vi "Data Recorder.vi"() -> ()   [LabVIEW 2021]
uses:
  Type Definitions/Data Frame.ctl
  Type Definitions/Data Frame Header.ctl
  Type Definitions/Payload Class.ctl
  Type Definitions/Device.ctl
  Type Definitions/Real Time Task Status.ctl
  Type Definitions/Enum - Data.ctl
  <vilib>/Platform/TimedLoop/XDataNode/timing_clust.ctl
  <vilib>/Platform/TimedLoop/XDataNode/nitl_modes.ctl
  <vilib>/Platform/TimedLoop/XDataNode/wakeup.ctl
  Type Definitions/Analog Data.ctl
  Type Definitions/Digital Input Data.ctl
  Type Definitions/Internet Connection Monitor.ctl
  Type Definitions/CPU Usage.ctl
  Type Definitions/Telemetry Recorder Status.ctl
  Type Definitions/Memory Monitor.ctl
  Type Definitions/Queue Monitor.ctl
  Type Definitions/RTOSMonitor.ctl
  Type Definitions/System Time.ctl
  <vilib>/platform/TimedLoop/XDataNode/XDataNode.xnode
  <vilib>/Platform/TimedLoop/XDataNode/XDNodeRunTimeDep.lvlib
panel:
  out "Frame":T1 {"CRC" format="%08x"; "Frame Header"."Options" format="%016b"; "Frame Header"."Time" format="%^<%I:%M:%S%3u %p\n%m/%d/%Y %Z>T"; "Frame Header"."Sync" format="%08x"}
  out "Payload ID":u16
  out "Numeric 2":i32
  out "error out 6":errorcluster
  out "Unhandled Data":T1 {"CRC" format="%08x"; "Frame Header"."Options" format="%016b"; "Frame Header"."Time" format="%^<%I:%M:%S%3u %p\n%m/%d/%Y %Z>T"; "Frame Header"."Sync" format="%08x"}
  out "error out 5":errorcluster
  out "error out 4":errorcluster
  out "error out 3":errorcluster
  out "error out 2":errorcluster
  out "output cluster":T5={"Task Name"="", "Priority"=100, "Processor"=-2, "Offset"=0, "Iteration Duration"=0, "Period"=0, "Finished Late"=FALSE}
  out "Numeric":i32
  out "error out":errorcluster
  out "data":T1 {"CRC" format="%08x"; "Frame Header"."Options" format="%016b"; "Frame Header"."Time" format="%^<%I:%M:%S%3u %p\n%m/%d/%Y %Z>T"; "Frame Header"."Sync" format="%08x"}
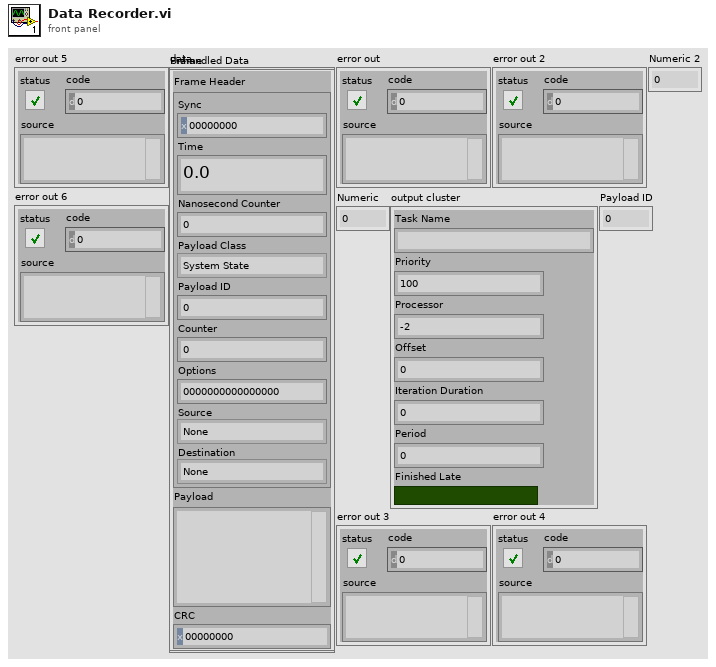
[diagram p1: front panel]
types:
  T1 = typedef "Data Frame.ctl" = cluster{"Frame Header":T2, "Payload":string, "CRC":u32}
  T2 = typedef "Data Frame Header.ctl" = cluster{"Sync":u32, "Time":dbl, "Nanosecond Counter":i64, "Payload Class":T3, "Payload ID":u16, "Counter":i32, "Options":u32, "Source":T4, "Destination":T4}
  T3 = typedef "Payload Class.ctl" = enum16{"System State", "Parameters", "Metadata", "Software Monitor", "Data", "Commands"}
  T4 = typedef "Device.ctl" = enum32{"None", "Exec", "Aux1", "Aux2", "Aux3"}
  T5 = typedef "Real Time Task Status.ctl" = cluster{"Task Name":string, "Priority":i32, "Processor":i32, "Offset":i64, "Iteration Duration":i64, "Period":i64, "Finished Late":bool}
  T6 = typedef "Enum - Data.ctl" = enum16{"Analog Input Data", "Notification Data", "Analog Output Data", "Digital Output Data", "Command Ack", "Digital Input Data", "GPS Solution Data"}
  T7 = enum16{"open", "replace", "create", "open or create", "replace or create", "replace or create with confirmation"}
  T8 = typedef "XDNodeRunTimeDep.lvlib/timing_clust.ctl" = cluster{"Expected End [f-1]":u64, "Actual End [f-1]":u64, "Finished Late? [f-1]":bool, "Expected End [i-1]":u64, "Actual End [i-1]":u64, "Finished Late? [i-1]":bool, "Expected Start [i]":u64, "Actual Start [i]":u64, "Expected Start [f]":u64, "Actual Start [f]":u64, "Source Name":string, "Structure Name":string, "Period":i64, "Deadline":i64, "Offset":i64, "Start":i64, "Priority":i32, "Timeout":i32, "Mode":T9, "Wakeup Reason":T10, "Error":errorcluster, "Source Type":string, "Secondary Source Type":string, "Global End Time":u64, "Global Start Time":u64, "Frame Duration":u64, "Iteration Duration":u64, "Assigned CPU":i32, "I/O Scan Engine Mode":u32}
  T9 = typedef "XDNodeRunTimeDep.lvlib/nitl_modes.ctl" = enum32{"No Change", "Process missed periods, maintain original phase", "Discard missed periods, maintain original phase", "Process missed periods, ignore original phase", "Discard missed periods, ignore original phase"}
  T10 = typedef "XDNodeRunTimeDep.lvlib/wakeup.ctl" = enum32{"Normal", "Aborted", "Asynchronous wakeup", "Timing source error", "Timed loop error", "Timeout"}
  T11 = typedef "Analog Data.ctl" = cluster{"Analog Data":sgl[][]}
  T12 = typedef "Digital Input Data.ctl" = cluster{"Digital Data":u64[][]}
  T13 = typedef "Internet Connection Monitor.ctl" = cluster{"Connected?":bool, "Ping Latency (uS)":i32, "Ping Address":string}
  T14 = typedef "CPU Usage.ctl" = cluster{"User CPU Usage":sgl, "System CPU Usage":sgl, "NIC CPU ":sgl, "IO CPU Usage":sgl, "IRQ CPU Usage":sgl, "SIRQ CPU Usage":sgl, "Idle CPU Time":sgl}
  T15 = typedef "Telemetry Recorder Status.ctl" = cluster{"Filepath":string, "File Size":i64, "Frame Count":i32, "Mean MB/hour":sgl}
  T16 = typedef "Memory Monitor.ctl" = cluster{"Total Memory":sgl, "Available Memory":sgl}
  T17 = typedef "Queue Monitor.ctl" = cluster{"Queue Name":string, "Max Queue Size":i32, "Pending Remove":i32, "Pending Insert":i32, "Elements in Queue":i32}
  T18 = typedef "RTOSMonitor.ctl" = cluster{"Task Name":string, "Priority":i32, "Processor":i32, "Offset":i64, "Min Duration":i64, "Mean Duration":i64, "Max Duration":i64, "Period":i64, "Late Iterations":i16, "Iteration Count":i32}
  T19 = typedef "System Time.ctl" = cluster{"System Clock":timestamp, "GPS Clock":timestamp, "Nanosecond Counter":i64, "GPS Status":enum8{"Initializing", "Normal", "Unable to get fix"}, "GPS Antenna Status":enum8{"Unknown", "Normal", "Absent", "Overcurrent"}, "GPS Satelites Available":u8, "GPS Time (ns)":u64, "GPS UTC Offset":i8, "GPS Time Offset":i32, "UTC Offset Valid":bool, "GPS Time Lock":bool}
  T20 = typedef "LVDateTimeRec.ctl" = cluster{"fractional second":dbl, "second":i32, "minute":i32, "hour":i32, "day of month":i32, "month":i32, "year":i32, "day of week":i32, "day of year":i32, "DST":i32}
  T21 = enum8{"Initializing", "Normal", "Unable to get fix"}
  T22 = enum8{"Unknown", "Normal", "Absent", "Overcurrent"}
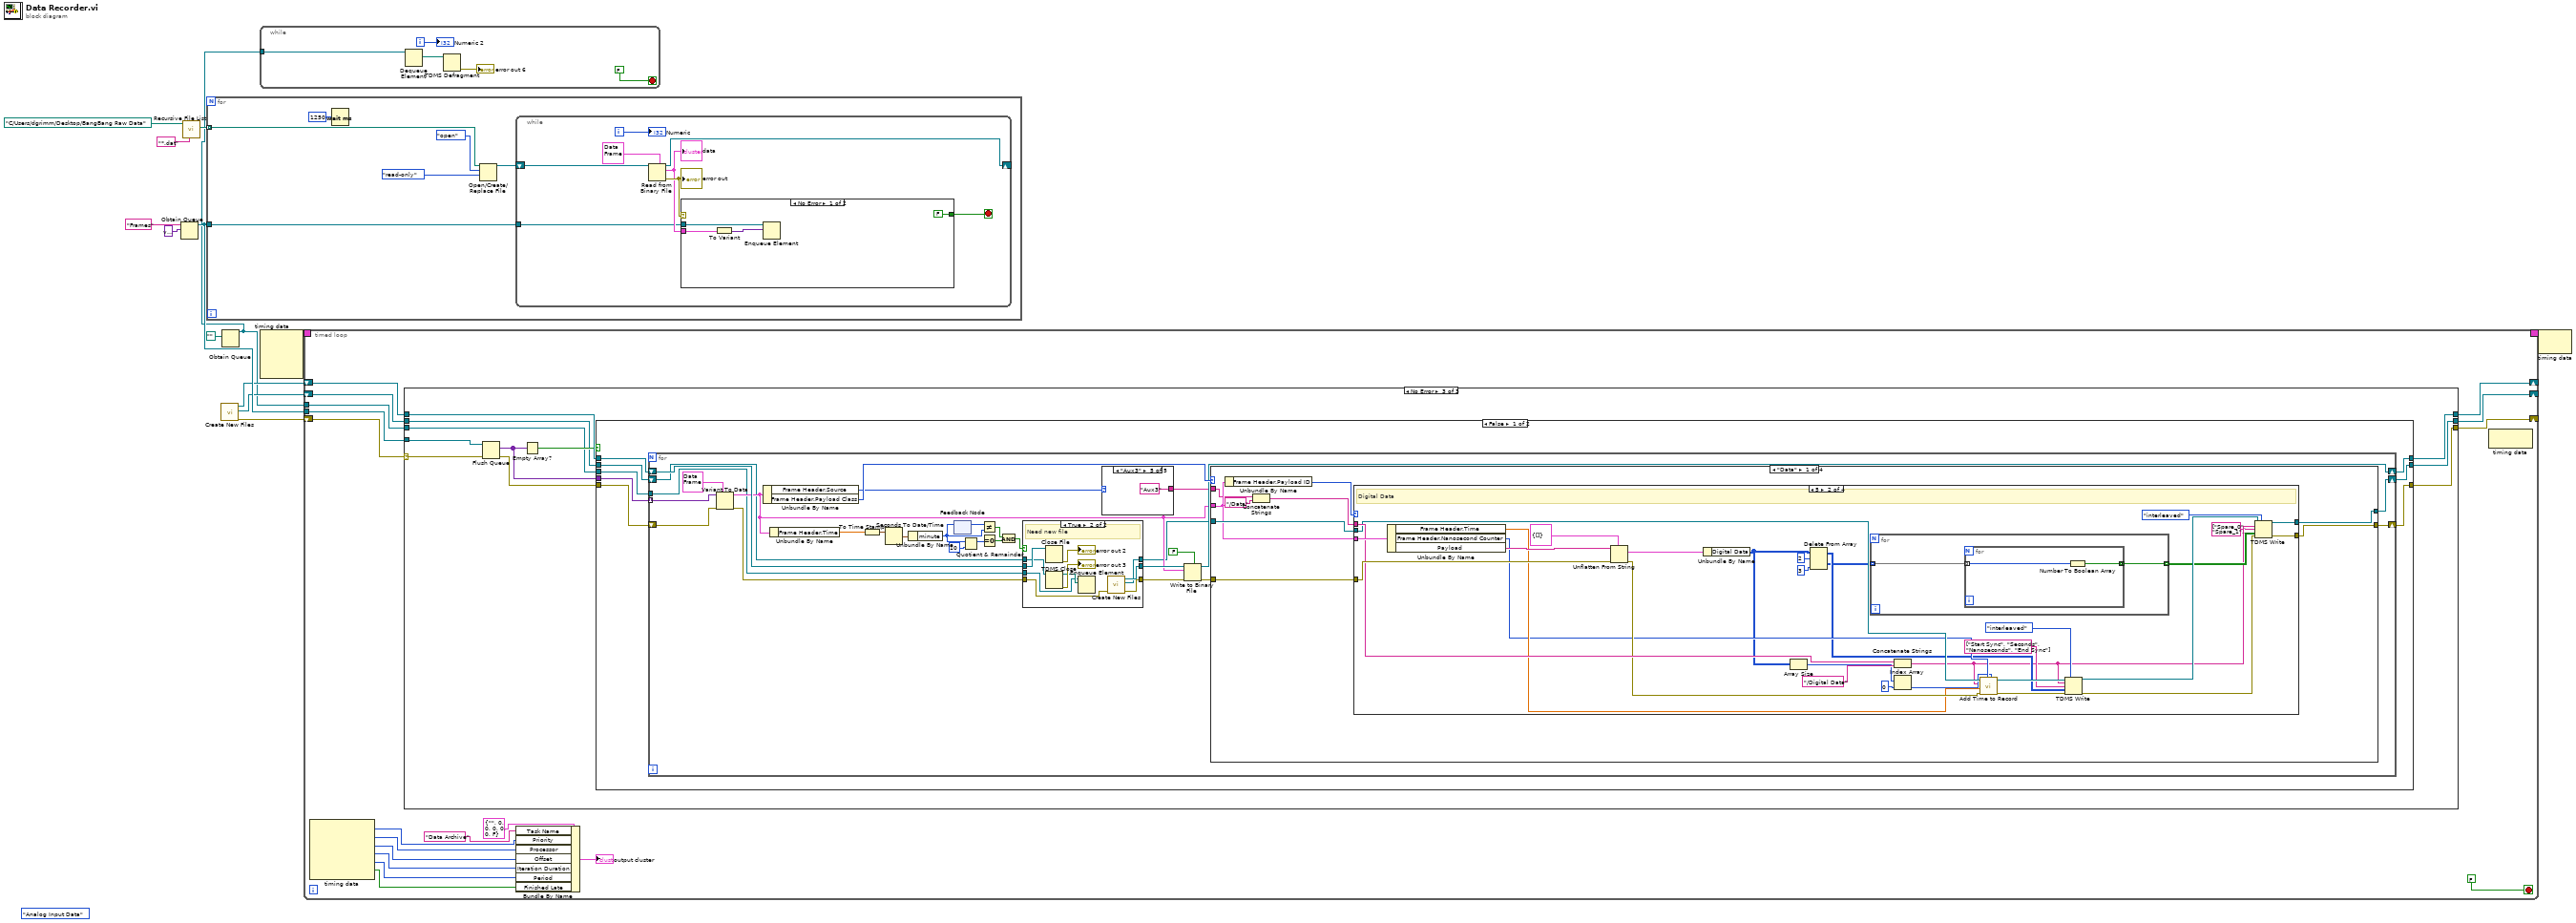
[diagram p0: block diagram]
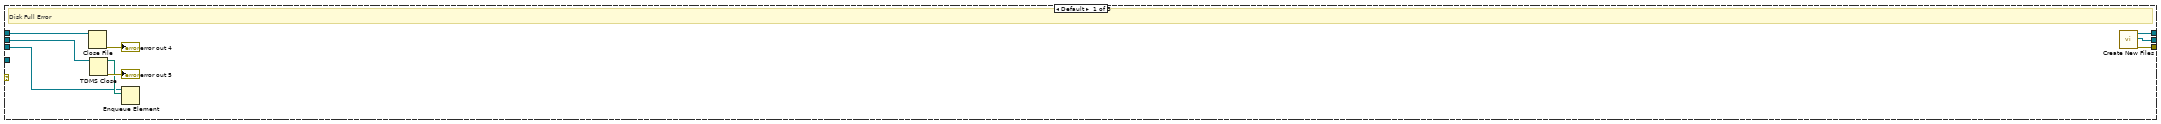
[diagram p2: hidden frame]
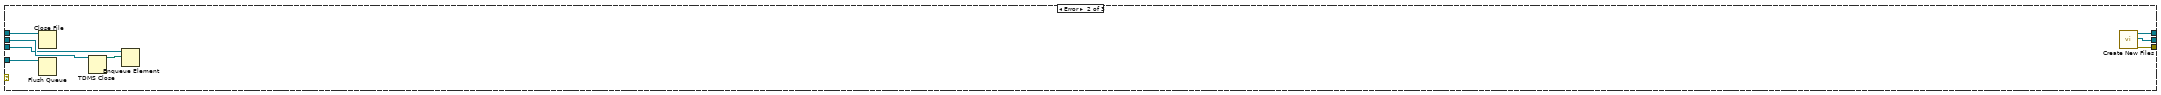
[diagram p3: hidden frame]
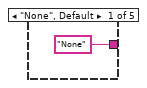
[diagram p4: hidden frame]
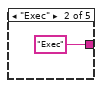
[diagram p5: hidden frame]
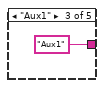
[diagram p6: hidden frame]
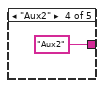
[diagram p7: hidden frame]
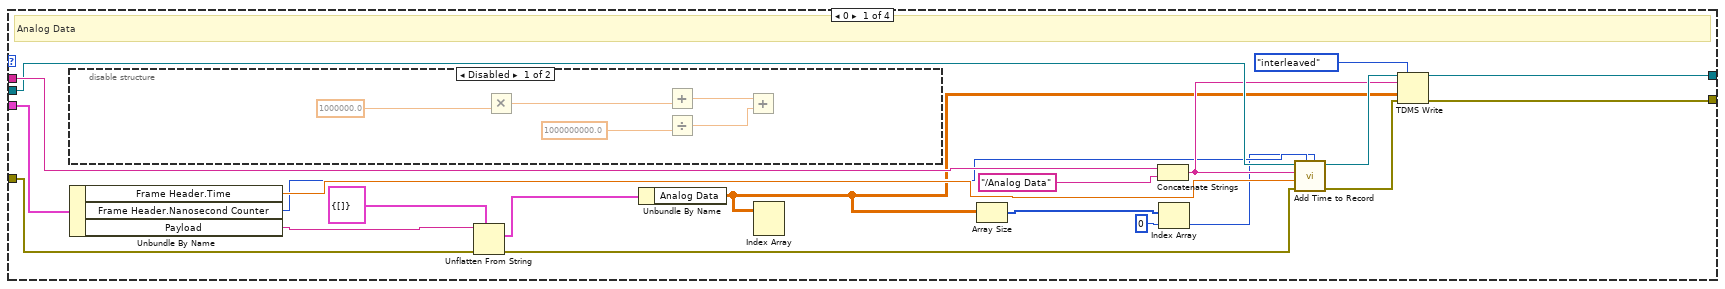
[diagram p9: hidden frame]
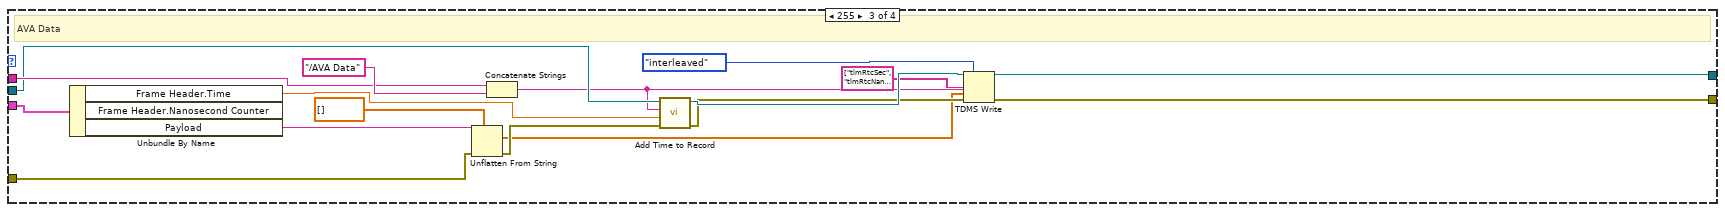
[diagram p11: hidden frame]
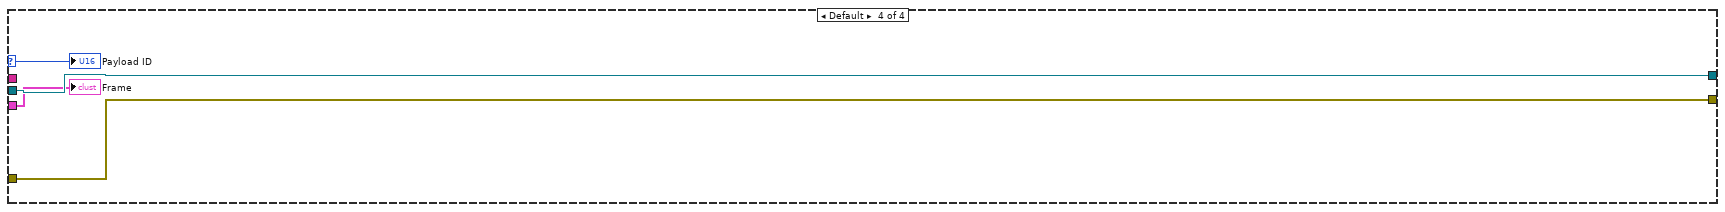
[diagram p12: hidden frame]
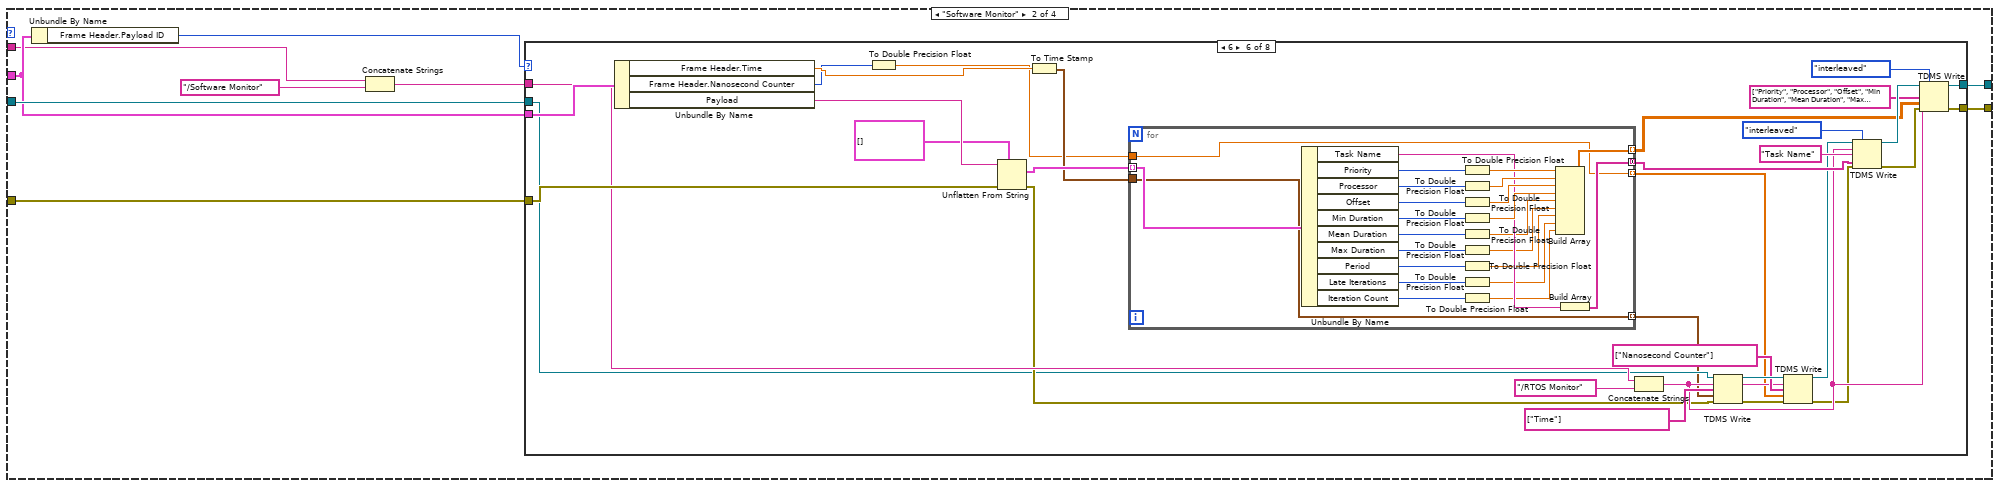
[diagram p13: hidden frame]
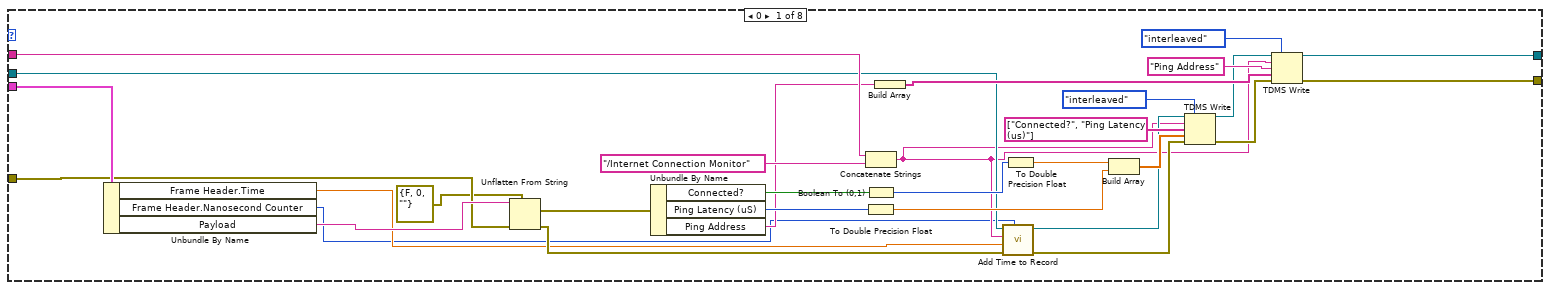
[diagram p14: hidden frame]
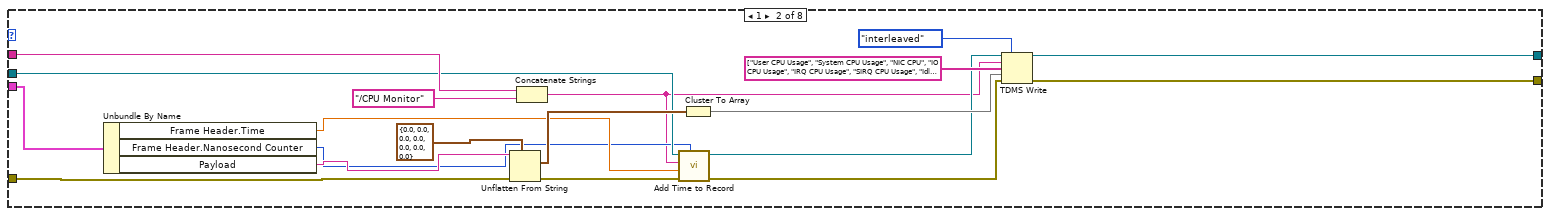
[diagram p15: hidden frame]
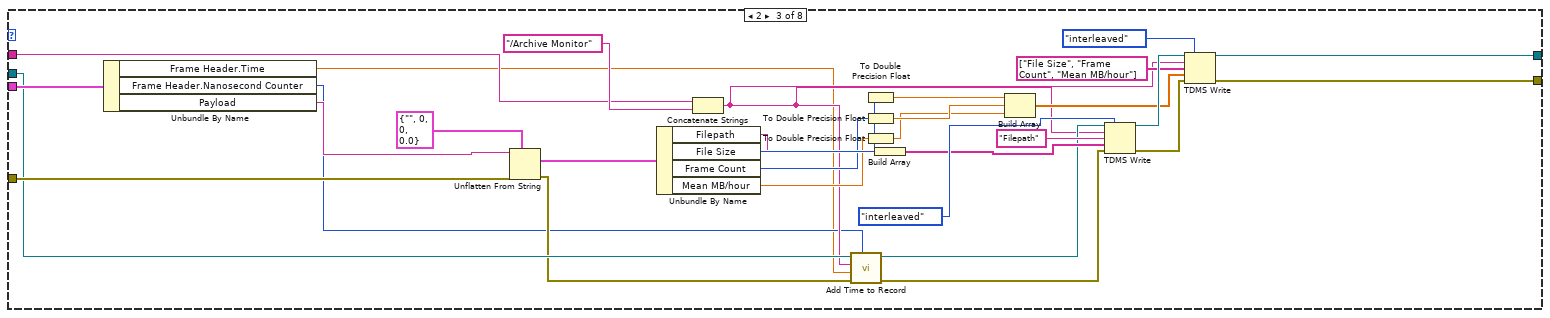
[diagram p16: hidden frame]
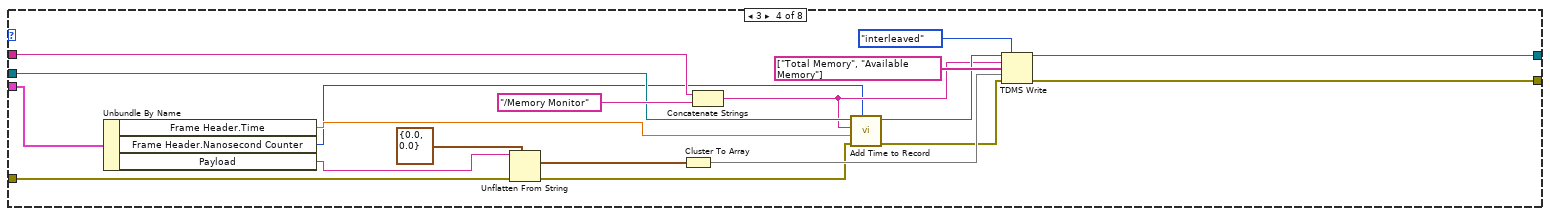
[diagram p17: hidden frame]
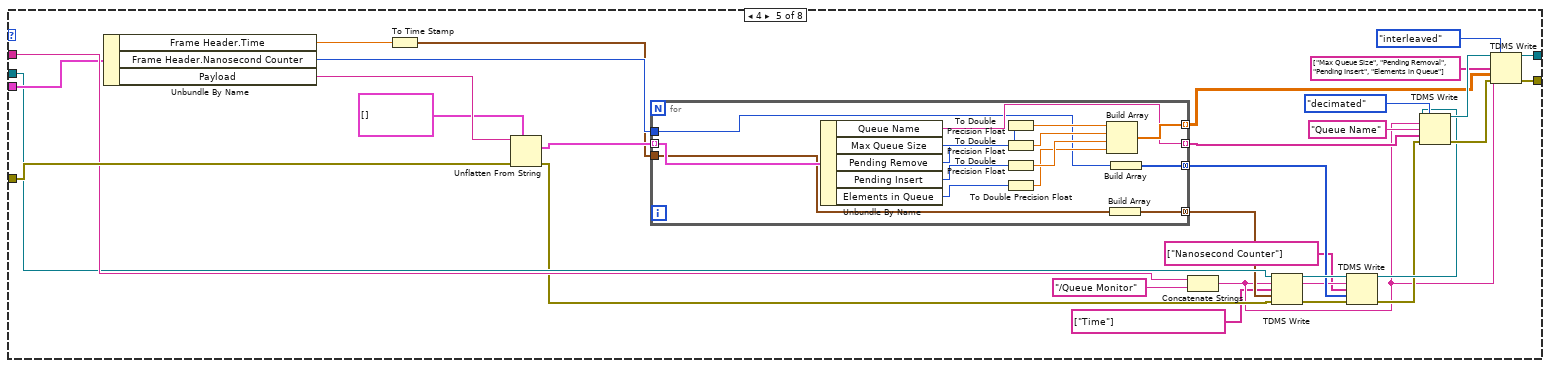
[diagram p18: hidden frame]
diagram:
  (unwired) Enum_-_Data."Analog Input Data" ("Data")
  n1 = Obtain Queue(name (unnamed)="Frames", element data type=variant) -> (queue out=w6:refnum<queue>)  [unwired: 3 in, 2 out]
  n2 = call <vilib>:"Recursive File List.vi"("pattern"="*.dat", "Folder Path"=path "C:/Users/dgrimm/Desktop/BangBang Raw Data" ("file (use dialog)")) -> ("All Files in Dir"=w12:path[])  [unwired: 5 in, 4 out]
  n3 = for {
    tunnel: w12 -> [w19] mode=indexing
    tunnel: w6 -> [w15]
    n4 = Wait (ms)(milliseconds to wait=u32 1250) -> ()  [unwired: 1 out]
    n5 = Open/Create/Replace File(file path (use dialog)=w19, operation (0:open)=T7."open", access (0:read/write)=enum16{"read/write", "read-only", "write-only"}."read-only") -> (refnum out=w16:refnum<file>)  [unwired: 3 in, 2 out]
    n6 = while {
      shift-right: [w25] -> _
      shift-left: w16 -> [w26]
      tunnel: w15 -> [w21]
      i -> [w20]
      stop <- w23 stop-if-true
      n7 = Read from Binary File(5:T1 {"Frame Header"={"Sync"=0, "Time"=0.0, "Nanosecond Counter"=0, "Payload Class"=enum."System State", "Payload ID"=0, "Counter"=0, "Options"=0, "Source"=enum."None", "Destination"=enum."None"}, "Payload"="", "CRC"=0} ("Frame"), 11:w26) -> (0:w24:errorcluster, 2:w22:T1, 3:w25:refnum<file>)  [unwired: 4 in, 1 out]
      "data" <- w22
      "error out" <- w24
      n8 = case shown="No Error" w24 {
        selector: w24 -> [_ w34]
        tunnel: [FALSE w32] -> w23
        tunnel: w22 -> [w30 _]
        tunnel: w21 -> [w28 _]
        frame No Error {
          n9 = To Variant(anything=w30) -> (Variant=w29:variant)
          n10 = Enqueue Element(queue=w28, element=w29) -> ()  [unwired: 2 in, 3 out]
        }
        frame Error {
          n11 = Unbundle By Name(w34) -> ("code"=w33:i32)
          n12 = case shown="0, Default" w33 {
            tunnel: [FALSE TRUE] -> w32
            frame 0, Default {
            }
            frame 4 {
            }
          }
        }
      }
      "Numeric" <- w20
    }
  }
  n13 = call "Create New Files.vi"() -> ("error out"=w4:errorcluster, "TDMS File Reference"=w3:refnum<k34>, "Binary File Reference"=w5:refnum<file>)  [unwired: 9 in]
  n14 = Obtain Queue(element data type=path "") -> (queue out=w1:refnum<queue>)  [unwired: 4 in, 2 out]
  n15 = while {
    tunnel: w1 -> [w40]
    i -> [w37]
    stop <- FALSE stop-if-true
    n16 = Dequeue Element(queue=w40) -> (element=w39:path)  [unwired: 2 in, 3 out]
    n17 = TDMS Defragment(7:w39) -> (0:→"error out 6":errorcluster)  [unwired: 1 in]
    "Numeric 2" <- w37
  }
  n18 = node-c288() -> (w8:T8)  [unwired: 4 in]
  n19 = timed-loop {
    tunnel: w6 -> [w59]
    shift-right: [w57] -> _
    shift-left: w4 -> [w54]
    shift-right: [w56] -> _
    shift-left: w5 -> [w55]
    timing: w8 -> [_]
    timing-out: [_] -> w7
    shift-right: [w53] -> _
    shift-left: w3 -> [w52]
    tunnel: w1 -> [w42]
    stop <- FALSE stop-if-true
    n20 = node-c288() -> (w50:i32, w49:i32, w48:i64, w47:i64, w46:i64, w45:bool)  [unwired: 1 in]
    n21 = case shown="No Error" w54 {
      selector: w54 -> [_ _ w93]
      tunnel: w59 -> [_ w83 w94]
      tunnel: [w74 w80 w90] -> w57
      tunnel: [w75 w82 w91] -> w56
      tunnel: w55 -> [w76 w84 w95]
      tunnel: [w73 w81 w86] -> w53
      tunnel: w52 -> [w72 w79 w87]
      tunnel: w42 -> [w68 w78 w85]
      frame Default {
        # "Disk Full Error"
        n22 = Close File(refnum=w76) -> (error out=→"error out 4":errorcluster)  [unwired: 1 in, 1 out]
        n23 = TDMS Close(11:w72) -> (0:→"error out 5":errorcluster, 3:w69:path)  [unwired: 1 in]
        n24 = Enqueue Element(queue=w68, element=w69) -> ()  [unwired: 2 in, 3 out]
        n25 = call "Create New Files.vi"() -> ("error out"=w74:errorcluster, "TDMS File Reference"=w73:refnum<k34>, "Binary File Reference"=w75:refnum<file>)  [unwired: 9 in]
      }
      frame Error {
        n26 = Close File(refnum=w84) -> ()  [unwired: 1 in, 2 out]
        n27 = Flush Queue(queue=w83) -> ()  [unwired: 1 in, 3 out]
        n28 = TDMS Close(11:w79) -> (3:w77:path)  [unwired: 1 in, 1 out]
        n29 = Enqueue Element(queue=w78, element=w77) -> ()  [unwired: 2 in, 3 out]
        n30 = call "Create New Files.vi"() -> ("error out"=w80:errorcluster, "TDMS File Reference"=w81:refnum<k34>, "Binary File Reference"=w82:refnum<file>)  [unwired: 9 in]
      }
      frame No Error {
        n31 = Flush Queue(queue=w94, error in (no error)=w93) -> (remaining elements=w89:variant[], error out=w92:errorcluster)  [unwired: 1 out]
        n32 = Empty Array?(array=w89) -> (empty?=w88:bool)
        n33 = case shown="False" w88 {
          tunnel: w95 -> [w97 w522]
          tunnel: w92 -> [w103 w523]
          tunnel: w89 -> [w102 _]
          tunnel: [w101 w522] -> w91
          tunnel: [w100 w523] -> w90
          tunnel: w87 -> [w99 w521]
          tunnel: [w98 w521] -> w86
          tunnel: w85 -> [w96 _]
          frame False {
            n34 = for {
              tunnel: w102 -> [w130] mode=indexing
              shift-right: [w107] -> w100
              shift-left: w103 -> [w131]
              shift-right: [w114] -> w101
              shift-left: w97 -> [w117]
              shift-right: [w111] -> w98
              shift-left: w99 -> [w109]
              tunnel: w96 -> [w104]
              n35 = Variant To Data(error in=w131, type=T1 {"Frame Header"={"Sync"=0, "Time"=0.0, "Nanosecond Counter"=0, "Payload Class"=enum."System State", "Payload ID"=0, "Counter"=0, "Options"=0, "Source"=enum."None", "Destination"=enum."None"}, "Payload"="", "CRC"=0} ("Frame"), Variant=w130) -> (data=w112:T1, error out=w118:errorcluster)
              n36 = Unbundle By Name(w112) -> ("Frame Header.Source"=w106:T4, "Frame Header.Payload Class"=w129:T3)
              n37 = Unbundle By Name(w112) -> ("Frame Header.Time"=w126:dbl)
              n38 = To Time Stamp(1:w126) -> (0:w127:timestamp)
              n39 = Seconds To Date/Time(time stamp (now)=w127) -> (date time rec=w119:T20)  [unwired: 1 in]
              n40 = Unbundle By Name(w119) -> ("minute"=w121:i32)
              n41 = feedback #1() -> (w122:i32)  [unwired: 1 in]
              n42 = feedback-in #1(w121) -> ()
              n43 = Quotient & Remainder(x=w121, y=10) -> (x-y*floor(x/y)=w124:i32)  [unwired: 1 out]
              n44 = Not Equal?(x=w122, y=w121) -> (x != y?=w120:bool)
              n45 = Equal To 0?(x=w124) -> (x = 0?=w123:bool)
              n46 = And(x=w120, y=w123) -> (x .and. y?=w128:bool)
              n47 = case shown="True" w128 {
                tunnel: [w139 w148] -> w113
                tunnel: w118 -> [w139 w149]
                tunnel: [w140 w147] -> w115
                tunnel: w117 -> [w140 w150]
                tunnel: [w138 w146] -> w110
                tunnel: w109 -> [w138 w145]
                tunnel: w104 -> [_ w141]
                frame False {
                  # "Current File is Good"
                }
                frame True {
                  # "Need new file"
                  n48 = Close File(refnum=w150) -> (error out=→"error out 2":errorcluster)  [unwired: 1 in, 1 out]
                  n49 = TDMS Close(11:w145) -> (0:→"error out 3":errorcluster, 3:w142:path)  [unwired: 1 in]
                  n50 = Enqueue Element(queue=w141, element=w142) -> ()  [unwired: 2 in, 3 out]
                  n51 = call "Create New Files.vi"("error in (no error)"=w149) -> ("error out"=w148:errorcluster, "TDMS File Reference"=w146:refnum<k34>, "Binary File Reference"=w147:refnum<file>)  [unwired: 8 in]
                }
              }
              n52 = case shown="\"Aux3\"" w106 {
                tunnel: ["None" "Exec" "Aux1" "Aux2" "Aux3"] -> w105
                frame "None", Default {
                }
                frame "Exec" {
                }
                frame "Aux1" {
                }
                frame "Aux2" {
                }
                frame "Aux3" {
                }
              }
              n53 = Write to Binary File(file (use dialog)=w115, data=w112, error in=w113, 5:FALSE ("prepend array or string size? (T)")) -> (refnum out=w114:refnum<file>, error out=w108:errorcluster)  [unwired: 2 in, 1 out]
              n54 = case shown="\"Data\"" w129 {
                tunnel: w112 -> [w154 w245 w459 w512]
                tunnel: w110 -> [w158 w249 w463 w516]
                tunnel: [w157 w248 w462 w515] -> w111
                tunnel: [w156 w247 w461 w514] -> w107
                tunnel: w108 -> [w155 w246 w460 w513]
                tunnel: w105 -> [w152 w243 w458 w511]
                frame "Data" {
                  n55 = Unbundle By Name(w154) -> ("Frame Header.Payload ID"=w159:u16)
                  n56 = Concatenate Strings(w152, "/Data" ("string")) -> (w151:string)
                  n57 = case shown="5" w159 {
                    selector: w159 -> [_ _ _ w239]
                    tunnel: w158 -> [w167 w208 w229 w241]
                    tunnel: [w180 w188 w237 w241] -> w157
                    tunnel: [w174 w189 w233 w240] -> w156
                    tunnel: w155 -> [w177 w214 w234 w240]
                    tunnel: w154 -> [w179 w216 w236 w238]
                    tunnel: w151 -> [w172 w210 w231 _]
                    frame 0 {
                      # "Analog Data"
                      n58 = disable-structure shown="Disabled" {
                        frame Disabled {
                          n59 = Multiply(y=1000000.0) -> (x*y=w184:dbl)  [unwired: 1 in]
                          n60 = Add(y=w184) -> (x+y=w181:dbl)  [unwired: 1 in]
                          n61 = Divide(y=1000000000.0) -> (x/y=w182:dbl)  [unwired: 1 in]
                          n62 = Add(x=w181, y=w182) -> ()  [unwired: 1 out]
                        }
                        frame Enabled {
                        }
                      }
                      n63 = Unbundle By Name(w179) -> ("Frame Header.Time"=w165:dbl, "Frame Header.Nanosecond Counter"=w164:i64, "Payload"=w178:string)
                      n64 = Unflatten From String(type=T11 {"Analog Data"=[]} ("Analog Data"), binary string=w178, error in (no error)=w177) -> (value=w175:T11, error out=w170:errorcluster)  [unwired: 2 in, 1 out]
                      n65 = Unbundle By Name(w175) -> ("Analog Data"=w163:sgl[][])
                      n66 = Index Array(array=w163) -> ()  [unwired: 2 in, 1 out]
                      n67 = Array Size(array=w163) -> (size(s)=w162:i32[])
                      n68 = Concatenate Strings(w172, "/Analog Data" ("string")) -> (w166:string)
                      n69 = Index Array(array=w162, index=0) -> (element=w160:i32)
                      n70 = call "Add Time to Record.vi"("Array Size"=w160, "Nanosecond Counter"=w164, "error in (no error)"=w170, "Time"=w165, "Group Name"=w166, "TDMS In"=w167) -> ("error out"=w169:errorcluster, "TDMS Out"=w168:refnum<k34>)  [unwired: 4 in]
                      n71 = TDMS Write(0:w168, 1:enum16{"decimated", "interleaved"}."interleaved" ("data layout (0:decimated)"), 5:w166, 9:w163, 11:w169) -> (4:w180:refnum<k34>, 15:w174:errorcluster)  [unwired: 1 in, 2 out]
                    }
                    frame 5 {
                      # "Digital Data"
                      n72 = Unbundle By Name(w216) -> ("Frame Header.Time"=w204:dbl, "Frame Header.Nanosecond Counter"=w203:i64, "Payload"=w215:string)
                      n73 = Unflatten From String(type=T12 {"Digital Data"=[]} ("Digital Input Data"), binary string=w215, error in (no error)=w214) -> (value=w213:T12, error out=w205:errorcluster)  [unwired: 2 in, 1 out]
                      n74 = Unbundle By Name(w213) -> ("Digital Data"=w196:u64[][])
                      n75 = Array Size(array=w196) -> (size(s)=w198:i32[])
                      n76 = Delete From Array(array=w196, length=2, index (col)=3 ("disabled index (col)")) -> (deleted portion=w194:u64[][], array with subset deleted=w199:u64[][])  [unwired: 1 in]
                      n77 = for {
                        tunnel: w194 -> [w218] mode=indexing
                        tunnel: [w217] -> w191 mode=indexing
                        n78 = for {
                          tunnel: w218 -> [w220] mode=indexing
                          tunnel: [w219] -> w217 mode=concatenating
                          n79 = Number To Boolean Array(number=w220) -> (Boolean array=w219:bool[])
                        }
                      }
                      n80 = Concatenate Strings(w210, "/Digital Data" ("string")) -> (w190:string)
                      n81 = Index Array(array=w198, index=0) -> (element=w195:i32)
                      n82 = call "Add Time to Record.vi"("Array Size"=w195, "Nanosecond Counter"=w203, "error in (no error)"=w205, "Time"=w204, "Group Name"=w190, "TDMS In"=w208) -> ("error out"=w206:errorcluster, "TDMS Out"=w207:refnum<k34>)  [unwired: 4 in]
                      n83 = TDMS Write(0:w207, 1:enum16{"decimated", "interleaved"}."interleaved" ("data layout (0:decimated)"), 5:w190, 7:string[] ["Start Sync", "Seconds", "Nanoseconds", "End Sync"] ("channel name(s) in (Untitled)"), 9:w199, 11:w206) -> (4:w193:refnum<k34>, 15:w192:errorcluster)  [unwired: 2 out]
                      n84 = TDMS Write(0:w193, 1:enum16{"decimated", "interleaved"}."interleaved" ("data layout (0:decimated)"), 5:w190, 7:string[] ["Spare_0", "Spare_1", "Spare_2", "Spare_3", "Spare_4", "Spare_5", "Spare_6", "Spare_7", "Spare_8", "Spare_9", "Spare_10", "Spare_11", "Spare_12", "Spare_13", "Spare_14", "Spare_15", "ROV-G0001_TLKBK CLOSED", "ROV-O0004_TLKBK CLOSED", "ROV-F0002_TLKBK CLOSED", "ROV-F0001_TLKBK CLOSED", "ROV-GN0002_TLKBK CLOSED", "ROV-GN0001_TLKBK CLOSED", "ROV-O0002_TLKBK CLOSED", "ROV-O0001_TLKBK CLOSED", "ROV-G0001_TLKBK OPENED", "ROV-O0004_TLKBK OPENED", "ROV-F0002_TLKBK OPENED", "ROV-F0001_TLKBK OPENED", "ROV-GN0002_TLKBK OPENED", "ROV-GN0001_TLKBK OPENED", "ROV-O0002_TLKBK OPENED", "ROV-O0001_TLKBK OPENED", "Spare_16", "Spare_17", "Spare_18", "Spare_19", "Spare_20", "Spare_21", "Spare_22", "Spare_23", "Spare_24", "Spare_25", "Spare_26", "Spare_27", "Spare_28", "Spare_29", "ROV-N0001_TLKBK CLOSED", "ROV-N0001_TLKBK OPENED", "Spare_30", "Spare_31", "Spare_32", "Spare_33", "Spare_34", "Spare_35", "Spare_36", "Spare_37", "Spare_38", "Spare_39", "Spare_40", "Spare_41", "Spare_42", "Spare_43", "Spare_44", "Spare_45", "OPVV-2", "OPVV-1", "HAFV", "FPVV-2", "FPVV-1", "ROV-N0002", "ROV-N0001", "ROV-G0001", "ROV-O0004", "ROV-A0003", "ROV-F0002", "ROV-F0001", "ROV-GN0002", "ROV-GN0001", "ROV-O0002", "ROV-O0001", "Spare_46", "Spare_47", "Spare_48", "Spare_49", "Spare_50", "Spare_51", "Spare_52", "Spare_53", "Spare_54", "Spare_55", "Spare_56", "Spare_57", "Spare_58", "Spare_59", "Spare_60", "Spare_61", "Spare_62", "Spare_63", "Spare_64", "Spare_65", "Spare_66", "Spare_67", "Spare_68", "Spare_69", "Spare_70", "Spare_71", "Spare_72", "Spare_73", "Spare_74", "Spare_75", "Spare_76", "HAOV", "Spare_77", "Spare_78", "Spare_79", "Spare_80", "Spare_81", "Spare_82", "Spare_83", "Spare_84", "Spare_85", "Spare_86", "Spare_87", "Spare_88", "Spare_89", "Spare_90", "Spare_91", "Spare_92"] ("Digital Signal Names"), 9:w191, 11:w192) -> (4:w188:refnum<k34>, 15:w189:errorcluster)  [unwired: 2 out]
                    }
                    frame 255 {
                      # "AVA Data"
                      n85 = Unbundle By Name(w236) -> ("Frame Header.Time"=w225:dbl, "Payload"=w235:string)  [unwired: 1 out]
                      n86 = Unflatten From String(type=dbl[] [], binary string=w235, error in (no error)=w234) -> (value=w222:dbl[], error out=w226:errorcluster)  [unwired: 2 in, 1 out]
                      n87 = Concatenate Strings(w231, "/AVA Data" ("string")) -> (w224:string)
                      n88 = call "Add Time to Record.vi"("error in (no error)"=w226, "Time"=w225, "Group Name"=w224, "TDMS In"=w229) -> ("error out"=w227:errorcluster, "TDMS Out"=w228:refnum<k34>)  [unwired: 6 in]
                      n89 = TDMS Write(0:w228, 1:enum16{"decimated", "interleaved"}."interleaved" ("data layout (0:decimated)"), 5:w224, 7:string[] ["tlmRtcSec", "tlmRtcNanoSec", "egseTlmFrames", "packetsRcvd", "packetsSent", "lostPacketErrors", "checksumErrors", "missedPackets", "cmdAccepted", "cmdRejected", "vMajor", "vMinor", "vRevision", "POT-1", "POT-2", "POT-3", "POI", "TOT", "TOI", "PFT-1", "PFT-2", "PFT-3", "PFI", "TFT", "TFI", "LoxInletPressEst", "FuelInletPressEst", "NPPT", "NPTC", "NFPT", "NFTC", "OBBPV-1_Cmd", "OBBPV-2_Cmd", "FBBPV-1_Cmd", "FBBPV-2_Cmd", "NVV_Cmd", "NIV_Cmd", "LoxAbortReason", "LoxAbortReasonOverPressure", "LoxAbortReasonVenting", "LoxAbortReasonSensDq", "FuelAbortReason", "FuelAbortReasonOverPressure", "FuelAbortReasonVenting", "FuelAbortReasonSensDq", "FrameCounter", "ClockSeconds", "ClockNanoseconds", "ApplicationState", "SoftwareVersionMajor", "SoftwareVersionMinor", "SoftwareVersionPatch", "LoxTankPressControlActive", "FuelTankPressControlActive", "CommandsAccepted", "CommandsRejected", "Padding_5", "Padding_6", "digitalRedline", "digitalInhibit", "digitalArm", "Padding_7", "ignitionSequenceStatus", "shutdownSequenceStatus", "testSequenceStatus", "CRC"] ("Telemetry Names"), 9:w222, 11:w227) -> (4:w237:refnum<k34>, 15:w233:errorcluster)  [unwired: 2 out]
                    }
                    frame Default {
                      "Payload ID" <- w239
                      "Frame" <- w238
                    }
                  }
                }
                frame "Software Monitor" {
                  n90 = Unbundle By Name(w245) -> ("Frame Header.Payload ID"=w250:u16)
                  n91 = Concatenate Strings(w243, "/Software Monitor" ("string")) -> (w242:string)
                  n92 = case shown="6" w250 {
                    tunnel: w249 -> [w257 w285 w306 w337 w363 w403 w453 w455]
                    tunnel: [w261 w299 w312 w342 w369 w416 w453 w455] -> w248
                    tunnel: [w259 w295 w310 w341 w372 w419 w452 w454] -> w247
                    tunnel: w246 -> [w278 w296 w328 w347 w379 w425 w452 w454]
                    tunnel: w245 -> [w280 w298 w330 w349 w364 w427 _ _]
                    tunnel: w242 -> [w275 w293 w326 w345 w377 w423 _ _]
                    frame 0 {
                      n93 = Unbundle By Name(w280) -> ("Frame Header.Time"=w253:dbl, "Frame Header.Nanosecond Counter"=w251:i64, "Payload"=w279:string)
                      n94 = Unflatten From String(type=T13 {"Connected?"=FALSE, "Ping Latency (uS)"=0, "Ping Address"=""} ("Internet Connection Monitor"), binary string=w279, error in (no error)=w278) -> (value=w277:T13, error out=w256:errorcluster)  [unwired: 2 in, 1 out]
                      n95 = Unbundle By Name(w277) -> ("Connected?"=w268:bool, "Ping Latency (uS)"=w270:i32, "Ping Address"=w265:string)
                      n96 = Concatenate Strings(w275, "/Internet Connection Monitor" ("string")) -> (w252:string)
                      n97 = Boolean To (0,1)(Boolean=w268) -> (0, 1=w272:i16)
                      n98 = To Double Precision Float(number=w270) -> (double precision float=w269:dbl)
                      n99 = Build Array(w265) -> (w264:string[])
                      n100 = call "Add Time to Record.vi"("Nanosecond Counter"=w251, "error in (no error)"=w256, "Time"=w253, "Group Name"=w252, "TDMS In"=w257) -> ("error out"=w254:errorcluster, "TDMS Out"=w255:refnum<k34>)  [unwired: 5 in]
                      n101 = To Double Precision Float(number=w272) -> (double precision float=w271:dbl)
                      n102 = Build Array(w271, w269) -> (w267:dbl[])
                      n103 = TDMS Write(0:w255, 1:enum16{"decimated", "interleaved"}."interleaved" ("data layout (0:decimated)"), 5:w252, 7:string[] ["Connected?", "Ping Latency (us)"] ("channel name(s) in (Untitled)"), 9:w267, 11:w254) -> (4:w262:refnum<k34>, 15:w260:errorcluster)  [unwired: 2 out]
                      n104 = TDMS Write(0:w262, 1:enum16{"decimated", "interleaved"}."interleaved" ("data layout (0:decimated)"), 5:w252, 7:"Ping Address" ("channel name(s) in (Untitled)"), 9:w264, 11:w260) -> (4:w261:refnum<k34>, 15:w259:errorcluster)  [unwired: 2 out]
                    }
                    frame 1 {
                      n105 = Unbundle By Name(w298) -> ("Frame Header.Time"=w283:dbl, "Frame Header.Nanosecond Counter"=w282:i64, "Payload"=w297:string)
                      n106 = Unflatten From String(type=T14 {"User CPU Usage"=0.0, "System CPU Usage"=0.0, "NIC CPU "=0.0, "IO CPU Usage"=0.0, "IRQ CPU Usage"=0.0, "SIRQ CPU Usage"=0.0, "Idle CPU Time"=0.0}, binary string=w297, error in (no error)=w296) -> (value=w290:T14, error out=w284:errorcluster)  [unwired: 2 in, 1 out]
                      n107 = Concatenate Strings(w293, "/CPU Monitor" ("string")) -> (w281:string)
                      n108 = call "Add Time to Record.vi"("Nanosecond Counter"=w282, "error in (no error)"=w284, "Time"=w283, "Group Name"=w281, "TDMS In"=w285) -> ("error out"=w286:errorcluster, "TDMS Out"=w287:refnum<k34>)  [unwired: 5 in]
                      n109 = Cluster To Array(cluster=w290) -> (array=w289:sgl[])
                      n110 = TDMS Write(0:w287, 1:enum16{"decimated", "interleaved"}."interleaved" ("data layout (0:decimated)"), 5:w281, 7:string[] ["User CPU Usage", "System CPU Usage", "NIC CPU", "IO CPU Usage", "IRQ CPU Usage", "SIRQ CPU Usage", "Idle CPU Time"] ("channel name(s) in (Untitled)"), 9:w289, 11:w286) -> (4:w299:refnum<k34>, 15:w295:errorcluster)  [unwired: 2 out]
                    }
                    frame 2 {
                      n111 = Unbundle By Name(w330) -> ("Frame Header.Time"=w300:dbl, "Frame Header.Nanosecond Counter"=w301:i64, "Payload"=w329:string)
                      n112 = Unflatten From String(type=T15 {"Filepath"="", "File Size"=0, "Frame Count"=0, "Mean MB/hour"=0.0}, binary string=w329, error in (no error)=w328) -> (value=w323:T15, error out=w304:errorcluster)  [unwired: 2 in, 1 out]
                      n113 = Unbundle By Name(w323) -> ("Filepath"=w319:string, "File Size"=w322:i64, "Frame Count"=w321:i32, "Mean MB/hour"=w320:sgl)
                      n114 = Concatenate Strings(w326, "/Archive Monitor" ("string")) -> (w302:string)
                      n115 = call "Add Time to Record.vi"("Nanosecond Counter"=w301, "error in (no error)"=w304, "Time"=w300, "Group Name"=w302, "TDMS In"=w306) -> ("error out"=w303:errorcluster, "TDMS Out"=w305:refnum<k34>)  [unwired: 5 in]
                      n116 = To Double Precision Float(number=w322) -> (double precision float=w318:dbl)
                      n117 = To Double Precision Float(number=w321) -> (double precision float=w317:dbl)
                      n118 = To Double Precision Float(number=w320) -> (double precision float=w316:dbl)
                      n119 = Build Array(w319) -> (w315:string[])
                      n120 = Build Array(w318, w317, w316) -> (w308:dbl[])
                      n121 = TDMS Write(0:w305, 1:enum16{"decimated", "interleaved"}."interleaved" ("data layout (0:decimated)"), 5:w302, 7:"Filepath", 9:w315, 11:w303) -> (4:w313:refnum<k34>, 15:w311:errorcluster)  [unwired: 2 out]
                      n122 = TDMS Write(0:w313, 1:enum16{"decimated", "interleaved"}."interleaved" ("data layout (0:decimated)"), 5:w302, 7:string[] ["File Size", "Frame Count", "Mean MB/hour"] ("channel name(s) in (Untitled)"), 9:w308, 11:w311) -> (4:w312:refnum<k34>, 15:w310:errorcluster)  [unwired: 2 out]
                    }
                    frame 3 {
                      n123 = Unbundle By Name(w349) -> ("Frame Header.Time"=w332:dbl, "Frame Header.Nanosecond Counter"=w331:i64, "Payload"=w348:string)
                      n124 = Unflatten From String(type=T16 {"Total Memory"=0.0, "Available Memory"=0.0}, binary string=w348, error in (no error)=w347) -> (value=w340:T16, error out=w335:errorcluster)  [unwired: 2 in, 1 out]
                      n125 = Cluster To Array(cluster=w340) -> (array=w339:sgl[])
                      n126 = Concatenate Strings(w345, "/Memory Monitor" ("string")) -> (w333:string)
                      n127 = call "Add Time to Record.vi"("Nanosecond Counter"=w331, "error in (no error)"=w335, "Time"=w332, "Group Name"=w333, "TDMS In"=w337) -> ("error out"=w334:errorcluster, "TDMS Out"=w336:refnum<k34>)  [unwired: 5 in]
                      n128 = TDMS Write(0:w336, 1:enum16{"decimated", "interleaved"}."interleaved" ("data layout (0:decimated)"), 5:w333, 7:string[] ["Total Memory", "Available Memory"] ("channel name(s) in (Untitled)"), 9:w339, 11:w334) -> (4:w342:refnum<k34>, 15:w341:errorcluster)  [unwired: 2 out]
                    }
                    frame 4 {
                      n129 = Unbundle By Name(w364) -> ("Frame Header.Time"=w352:dbl, "Frame Header.Nanosecond Counter"=w355:i64, "Payload"=w380:string)
                      n130 = To Time Stamp(1:w352) -> (0:w351:timestamp)
                      n131 = Unflatten From String(type=T17[] [] ("cluster"), binary string=w380, error in (no error)=w379) -> (value=w374:T17[], error out=w360:errorcluster)  [unwired: 2 in, 1 out]
                      n132 = for {
                        tunnel: w374 -> [w395] mode=indexing
                        tunnel: [w386] -> w368 mode=indexing
                        tunnel: [w385] -> w366 mode=indexing
                        tunnel: [w383] -> w357 mode=concatenating
                        tunnel: w351 -> [w384]
                        tunnel: [w381] -> w356 mode=concatenating
                        tunnel: w355 -> [w382]
                        n133 = Unbundle By Name(w395) -> ("Queue Name"=w385:string, "Max Queue Size"=w394:i32, "Pending Remove"=w393:i32, "Pending Insert"=w392:i32, "Elements in Queue"=w391:i32)
                        n134 = To Double Precision Float(number=w394) -> (double precision float=w390:dbl)
                        n135 = To Double Precision Float(number=w393) -> (double precision float=w389:dbl)
                        n136 = To Double Precision Float(number=w392) -> (double precision float=w388:dbl)
                        n137 = To Double Precision Float(number=w391) -> (double precision float=w387:dbl)
                        n138 = Build Array(w390, w389, w388, w387) -> (w386:dbl[])
                        n139 = Build Array(w384) -> (w383:timestamp[])
                        n140 = Build Array(w382) -> (w381:i64[])
                      }
                      n141 = Concatenate Strings(w377, "/Queue Monitor" ("string")) -> (w354:string)
                      n142 = TDMS Write(0:w363, 5:w354, 7:string[] ["Time"] ("channel name(s) in (Untitled)"), 9:w357, 11:w360) -> (4:w362:refnum<k34>, 15:w359:errorcluster)  [unwired: 1 in, 2 out]
                      n143 = TDMS Write(0:w362, 5:w354, 7:string[] ["Nanosecond Counter"] ("channel name(s) in (Untitled)"), 9:w356, 11:w359) -> (4:w361:refnum<k34>, 15:w358:errorcluster)  [unwired: 1 in, 2 out]
                      n144 = TDMS Write(0:w361, 1:enum16{"decimated", "interleaved"}."decimated" ("data layout (0:decimated)"), 5:w354, 7:"Queue Name", 9:w366, 11:w358) -> (4:w371:refnum<k34>, 15:w373:errorcluster)  [unwired: 2 out]
                      n145 = TDMS Write(0:w371, 1:enum16{"decimated", "interleaved"}."interleaved" ("data layout (0:decimated)"), 5:w354, 7:string[] ["Max Queue Size", "Pending Removal", "Pending Insert", "Elements in Queue"] ("channel name(s) in (Untitled)"), 9:w368, 11:w373) -> (4:w369:refnum<k34>, 15:w372:errorcluster)  [unwired: 2 out]
                    }
                    frame 6 {
                      n146 = Unbundle By Name(w427) -> ("Frame Header.Time"=w401:dbl, "Frame Header.Nanosecond Counter"=w400:i64, "Payload"=w426:string)
                      n147 = To Double Precision Float(number=w400) -> (double precision float=w396:dbl)
                      n148 = Unflatten From String(type=T18[] [] ("cluster"), binary string=w426, error in (no error)=w425) -> (value=w421:T18[], error out=w405:errorcluster)  [unwired: 2 in, 1 out]
                      n149 = To Time Stamp(1:w401) -> (0:w398:timestamp)
                      n150 = for {
                        tunnel: w421 -> [w451] mode=indexing
                        tunnel: [w442] -> w415 mode=indexing
                        tunnel: [w440] -> w413 mode=concatenating
                        tunnel: [w429] -> w399 mode=indexing
                        tunnel: w398 -> [w429]
                        tunnel: [w428] -> w397 mode=indexing
                        tunnel: w396 -> [w428]
                        n151 = Unbundle By Name(w451) -> ("Task Name"=w441:string, "Priority"=w450:i32, "Processor"=w449:i32, "Offset"=w448:i64, "Min Duration"=w447:i64, "Mean Duration"=w439:i64, "Max Duration"=w438:i64, "Period"=w437:i64, "Late Iterations"=w435:i16, "Iteration Count"=w436:i32)
                        n152 = To Double Precision Float(number=w450) -> (double precision float=w446:dbl)
                        n153 = To Double Precision Float(number=w449) -> (double precision float=w445:dbl)
                        n154 = To Double Precision Float(number=w448) -> (double precision float=w444:dbl)
                        n155 = To Double Precision Float(number=w447) -> (double precision float=w443:dbl)
                        n156 = To Double Precision Float(number=w439) -> (double precision float=w434:dbl)
                        n157 = To Double Precision Float(number=w438) -> (double precision float=w433:dbl)
                        n158 = To Double Precision Float(number=w437) -> (double precision float=w432:dbl)
                        n159 = To Double Precision Float(number=w435) -> (double precision float=w431:dbl)
                        n160 = To Double Precision Float(number=w436) -> (double precision float=w430:dbl)
                        n161 = Build Array(w446, w445, w444, w443, w434, w433, w432, w431, w430) -> (w442:dbl[])
                        n162 = Build Array(w441) -> (w440:string[])
                      }
                      n163 = Concatenate Strings(w423, "/RTOS Monitor" ("string")) -> (w406:string)
                      n164 = TDMS Write(0:w403, 5:w406, 7:string[] ["Time"] ("channel name(s) in (Untitled)"), 9:w399, 11:w405) -> (4:w410:refnum<k34>, 15:w409:errorcluster)  [unwired: 1 in, 2 out]
                      n165 = TDMS Write(0:w410, 5:w406, 7:string[] ["Nanosecond Counter"] ("channel name(s) in (Untitled)"), 9:w397, 11:w409) -> (4:w402:refnum<k34>, 15:w404:errorcluster)  [unwired: 1 in, 2 out]
                      n166 = TDMS Write(0:w402, 1:enum16{"decimated", "interleaved"}."interleaved" ("data layout (0:decimated)"), 5:w406, 7:"Task Name", 9:w413, 11:w404) -> (4:w418:refnum<k34>, 15:w420:errorcluster)  [unwired: 2 out]
                      n167 = TDMS Write(0:w418, 1:enum16{"decimated", "interleaved"}."interleaved" ("data layout (0:decimated)"), 5:w406, 7:string[] ["Priority", "Processor", "Offset", "Min Duration", "Mean Duration", "Max Duration", "Period", "Late Iterations", "Iteration Count"] ("channel name(s) in (Untitled)"), 9:w415, 11:w420) -> (4:w416:refnum<k34>, 15:w419:errorcluster)  [unwired: 2 out]
                    }
                    frame 5 {
                    }
                    frame Default {
                    }
                  }
                }
                frame "System State" {
                  n168 = Unbundle By Name(w459) -> ("Frame Header.Payload ID"=w464:u16)
                  n169 = Concatenate Strings(w458, "/System State" ("string")) -> (w456:string)
                  n170 = case shown="0" w464 {
                    tunnel: w463 -> [w506 w508]
                    tunnel: [w494 w508] -> w462
                    tunnel: [w492 w507] -> w461
                    tunnel: w460 -> [w503 w507]
                    tunnel: w459 -> [w505 _]
                    tunnel: w456 -> [w497 _]
                    frame 0 {
                      n171 = Unbundle By Name(w505) -> ("Payload"=w504:string)
                      n172 = Unflatten From String(type=T19 {"System Clock"=timestamp(0 s since 1904-01-01), "GPS Clock"=timestamp(0 s since 1904-01-01), "Nanosecond Counter"=0, "GPS Status"=enum."Initializing", "GPS Antenna Status"=enum."Unknown", "GPS Satelites Available"=0, "GPS Time (ns)"=0, "GPS UTC Offset"=0, "GPS Time Offset"=0, "UTC Offset Valid"=FALSE, "GPS Time Lock"=FALSE}, binary string=w504, error in (no error)=w503) -> (value=w500:T19, error out=w502:errorcluster)  [unwired: 2 in, 1 out]
                      n173 = Unbundle By Name(w500) -> ("System Clock"=w499:timestamp, "GPS Clock"=w498:timestamp, "Nanosecond Counter"=w491:i64, "GPS Status"=w488:T21, "GPS Antenna Status"=w487:T22, "GPS Satelites Available"=w484:u8, "GPS Time (ns)"=w483:u64, "GPS UTC Offset"=w480:i8, "GPS Time Offset"=w479:i32, "UTC Offset Valid"=w475:bool, "GPS Time Lock"=w473:bool)
                      n174 = Build Array(w499, w498) -> (w469:timestamp[])
                      n175 = Boolean To (0,1)(Boolean=w475) -> (0, 1=w477:i16)
                      n176 = Boolean To (0,1)(Boolean=w473) -> (0, 1=w476:i16)
                      n177 = Concatenate Strings(w497, "/System Time" ("string")) -> (w471:string)
                      n178 = To Double Precision Float(number=w480) -> (double precision float=w481:dbl)
                      n179 = To Double Precision Float(number=w479) -> (double precision float=w478:dbl)
                      n180 = TDMS Write(0:w506, 1:enum16{"decimated", "interleaved"}."interleaved" ("data layout (0:decimated)"), 5:w471, 7:string[] ["System Clock", "GPS Clock"] ("channel name(s) in (Untitled)"), 9:w469, 11:w502) -> (4:w495:refnum<k34>, 15:w493:errorcluster)  [unwired: 2 out]
                      n181 = To Double Precision Float(number=w491) -> (double precision float=w490:dbl)
                      n182 = To Double Precision Float(number=w488) -> (double precision float=w489:dbl)
                      n183 = To Double Precision Float(number=w487) -> (double precision float=w486:dbl)
                      n184 = To Double Precision Float(number=w484) -> (double precision float=w485:dbl)
                      n185 = To Double Precision Float(number=w483) -> (double precision float=w482:dbl)
                      n186 = To Double Precision Float(number=w477) -> (double precision float=w474:dbl)
                      n187 = To Double Precision Float(number=w476) -> (double precision float=w467:dbl)
                      n188 = Build Array(w490, w489, w486, w485, w482, w481, w478, w474, w467) -> (w472:dbl[])
                      n189 = TDMS Write(0:w495, 1:enum16{"decimated", "interleaved"}."interleaved" ("data layout (0:decimated)"), 5:w471, 7:string[] ["Nanosecond Counter", "GPS Status", "GPS Antenna Status", "GPS Satelites Available", "GPS Time (ns)", "GPS UTC Offset", "GPS Time Offset", "UTC Offset Valid", "GPS Time Lock"] ("channel name(s) in (Untitled)"), 9:w472, 11:w493) -> (4:w494:refnum<k34>, 15:w492:errorcluster)  [unwired: 2 out]
                    }
                    frame Default {
                    }
                  }
                }
                frame Default {
                  n190 = Unbundle By Name(w512) -> ("Frame Header.Payload ID"=w517:u16)
                  n191 = Concatenate Strings(w511, "/Default" ("string")) -> (w509:string)
                  n192 = case shown="Default" w517 {
                    tunnel: w516 -> [w520]
                    tunnel: [w520] -> w515
                    tunnel: [w519] -> w514
                    tunnel: w513 -> [w519]
                    tunnel: w512 -> [w518]
                    tunnel: w509 -> [_]
                    frame Default {
                      "Unhandled Data" <- w518
                    }
                  }
                }
              }
            }
          }
          frame True {
            # "Empty archive queue"
          }
        }
      }
    }
    n193 = Bundle By Name(cluster=T5 {"Task Name"="", "Priority"=0, "Processor"=0, "Offset"=0, "Iteration Duration"=0, "Period"=0, "Finished Late"=FALSE} ("Cluster"), "Task Name"="Data Archive", "Priority"=w50, "Processor"=w49, "Offset"=w48, "Iteration Duration"=w47, "Period"=w46, "Finished Late"=w45) -> (→"output cluster":T5)
    n194 = node-c288() -> ()  [unwired: 1 in, 1 out]
  }
  n195 = node-c288(w7) -> ()  [unwired: 1 out]
